vi "Main.vi"() -> ()   [LabVIEW 2021] (continued)
                    n838 = invoke on="控件配置文件" class="Tbl (严格)" method="Set Cell Value"("X Index"=0 ("X索引"), "Y Index"=w1041, "Value"=w1046) -> ()  [unwired: 3 in, 6 out]
                  }
                  frame "关联到曲线29" {
                    w1052 = T9 58 items=["刷新间隔", "波特率", "布尔1设置项", "布尔2设置项", "布尔3设置项", "布尔4设置项", "布尔5设置项", "布尔6设置项", "布尔7设置项", "布尔8设置项", "显控1设置", "显控2设置", "显控3设置", "显控4设置", "显控5设置", "显控6设置", "显控7设置", "显控8设置", "显控9设置", "显控10设置", "显控11设置", "显控12设置", "设控1设置", "设控2设置", "设控3设置", "设控4设置", "设控5设置", "设控6设置", "设控7设置", "设控8设置", "曲线1设置", "曲线2设置", "曲线3设置", "曲线4设置", "曲线5设置", "曲线6设置", "曲线7设置", "曲线8设置", "曲线9设置", "曲线10设置", "曲线11设置", "曲线12设置", "曲线13设置", "曲线14设置", "曲线15设置", "曲线16设置", "曲线17设置", "曲线18设置", "曲线19设置", "曲线20设置", "曲线21设置", "曲线22设置", "曲线23设置", "曲线24设置", "曲线25设置", "曲线26设置", "曲线27设置", "曲线28设置", "曲线29设置", "曲线30设置", "曲线31设置", "曲线32设置", "曲线33设置", "曲线34设置", "曲线35设置", "曲线36设置", "曲线37设置", "曲线38设置", "曲线39设置", "曲线40设置", "曲线41设置", "曲线42设置", "曲线43设置", "曲线44设置", "曲线45设置", "曲线46设置", "曲线47设置", "曲线48设置", "曲线49设置", "曲线50设置", "曲线51设置", "曲线52设置", "曲线53设置", "曲线54设置", "曲线55设置", "曲线56设置", "曲线57设置", "曲线58设置", "曲线59设置", "曲线60设置", "曲线61设置", "曲线62设置", "曲线63设置", "曲线64设置", "ID值", "数据模式"] ("DataInitDef")
                    n839 = property on="表格" class="Tbl (严格)"() -> ("Selection Start"=w1062:T1)  [unwired: 2 in, 2 out]
                    n840 = Unbundle By Name(w1062) -> ("Row"=w1060:i32)
                    n841 = property on="表格" class="Tbl (严格)"() -> ("Value"=w1061:string[][])  [unwired: 2 in, 2 out]
                    n842 = Number To Decimal String(number=w1060) -> (decimal integer string=w1059:string)  [unwired: 1 in]
                    n843 = Index Array(array=w1061, index (row)=w1060, index (col)=0 ("禁用的索引 (列)")) -> (element=w1058:string)
                    n844 = String Subset(string=w1058, length (rest)=16 ("长度（剩余）")) -> (substring=w1057:string)  [unwired: 1 in]
                    n845 = property on="曲线29设置" class="Str"("Val(Sgnl)"=w1057) -> ()  [unwired: 2 in, 2 out]
                    n846 = invoke on="控件配置文件" class="Tbl (严格)" method="Set Cell Value"("X Index"=1 ("X索引"), "Y Index"=w1052, "Value"=w1059) -> ()  [unwired: 3 in, 6 out]
                    n847 = invoke on="控件配置文件" class="Tbl (严格)" method="Set Cell Value"("X Index"=0 ("X索引"), "Y Index"=w1052, "Value"=w1057) -> ()  [unwired: 3 in, 6 out]
                  }
                  frame "关联到曲线30" {
                    w1063 = T9 59 items=["刷新间隔", "波特率", "布尔1设置项", "布尔2设置项", "布尔3设置项", "布尔4设置项", "布尔5设置项", "布尔6设置项", "布尔7设置项", "布尔8设置项", "显控1设置", "显控2设置", "显控3设置", "显控4设置", "显控5设置", "显控6设置", "显控7设置", "显控8设置", "显控9设置", "显控10设置", "显控11设置", "显控12设置", "设控1设置", "设控2设置", "设控3设置", "设控4设置", "设控5设置", "设控6设置", "设控7设置", "设控8设置", "曲线1设置", "曲线2设置", "曲线3设置", "曲线4设置", "曲线5设置", "曲线6设置", "曲线7设置", "曲线8设置", "曲线9设置", "曲线10设置", "曲线11设置", "曲线12设置", "曲线13设置", "曲线14设置", "曲线15设置", "曲线16设置", "曲线17设置", "曲线18设置", "曲线19设置", "曲线20设置", "曲线21设置", "曲线22设置", "曲线23设置", "曲线24设置", "曲线25设置", "曲线26设置", "曲线27设置", "曲线28设置", "曲线29设置", "曲线30设置", "曲线31设置", "曲线32设置", "曲线33设置", "曲线34设置", "曲线35设置", "曲线36设置", "曲线37设置", "曲线38设置", "曲线39设置", "曲线40设置", "曲线41设置", "曲线42设置", "曲线43设置", "曲线44设置", "曲线45设置", "曲线46设置", "曲线47设置", "曲线48设置", "曲线49设置", "曲线50设置", "曲线51设置", "曲线52设置", "曲线53设置", "曲线54设置", "曲线55设置", "曲线56设置", "曲线57设置", "曲线58设置", "曲线59设置", "曲线60设置", "曲线61设置", "曲线62设置", "曲线63设置", "曲线64设置", "ID值", "数据模式"] ("DataInitDef")
                    n848 = property on="表格" class="Tbl (严格)"() -> ("Selection Start"=w1073:T1)  [unwired: 2 in, 2 out]
                    n849 = Unbundle By Name(w1073) -> ("Row"=w1071:i32)
                    n850 = property on="表格" class="Tbl (严格)"() -> ("Value"=w1072:string[][])  [unwired: 2 in, 2 out]
                    n851 = Number To Decimal String(number=w1071) -> (decimal integer string=w1070:string)  [unwired: 1 in]
                    n852 = Index Array(array=w1072, index (row)=w1071, index (col)=0 ("禁用的索引 (列)")) -> (element=w1069:string)
                    n853 = String Subset(string=w1069, length (rest)=16 ("长度（剩余）")) -> (substring=w1068:string)  [unwired: 1 in]
                    n854 = property on="曲线30设置" class="Str"("Val(Sgnl)"=w1068) -> ()  [unwired: 2 in, 2 out]
                    n855 = invoke on="控件配置文件" class="Tbl (严格)" method="Set Cell Value"("X Index"=1 ("X索引"), "Y Index"=w1063, "Value"=w1070) -> ()  [unwired: 3 in, 6 out]
                    n856 = invoke on="控件配置文件" class="Tbl (严格)" method="Set Cell Value"("X Index"=0 ("X索引"), "Y Index"=w1063, "Value"=w1068) -> ()  [unwired: 3 in, 6 out]
                  }
                  frame "关联到曲线31" {
                    w1074 = T9 60 items=["刷新间隔", "波特率", "布尔1设置项", "布尔2设置项", "布尔3设置项", "布尔4设置项", "布尔5设置项", "布尔6设置项", "布尔7设置项", "布尔8设置项", "显控1设置", "显控2设置", "显控3设置", "显控4设置", "显控5设置", "显控6设置", "显控7设置", "显控8设置", "显控9设置", "显控10设置", "显控11设置", "显控12设置", "设控1设置", "设控2设置", "设控3设置", "设控4设置", "设控5设置", "设控6设置", "设控7设置", "设控8设置", "曲线1设置", "曲线2设置", "曲线3设置", "曲线4设置", "曲线5设置", "曲线6设置", "曲线7设置", "曲线8设置", "曲线9设置", "曲线10设置", "曲线11设置", "曲线12设置", "曲线13设置", "曲线14设置", "曲线15设置", "曲线16设置", "曲线17设置", "曲线18设置", "曲线19设置", "曲线20设置", "曲线21设置", "曲线22设置", "曲线23设置", "曲线24设置", "曲线25设置", "曲线26设置", "曲线27设置", "曲线28设置", "曲线29设置", "曲线30设置", "曲线31设置", "曲线32设置", "曲线33设置", "曲线34设置", "曲线35设置", "曲线36设置", "曲线37设置", "曲线38设置", "曲线39设置", "曲线40设置", "曲线41设置", "曲线42设置", "曲线43设置", "曲线44设置", "曲线45设置", "曲线46设置", "曲线47设置", "曲线48设置", "曲线49设置", "曲线50设置", "曲线51设置", "曲线52设置", "曲线53设置", "曲线54设置", "曲线55设置", "曲线56设置", "曲线57设置", "曲线58设置", "曲线59设置", "曲线60设置", "曲线61设置", "曲线62设置", "曲线63设置", "曲线64设置", "ID值", "数据模式"] ("DataInitDef")
                    n857 = property on="表格" class="Tbl (严格)"() -> ("Selection Start"=w1084:T1)  [unwired: 2 in, 2 out]
                    n858 = Unbundle By Name(w1084) -> ("Row"=w1082:i32)
                    n859 = property on="表格" class="Tbl (严格)"() -> ("Value"=w1083:string[][])  [unwired: 2 in, 2 out]
                    n860 = Number To Decimal String(number=w1082) -> (decimal integer string=w1081:string)  [unwired: 1 in]
                    n861 = Index Array(array=w1083, index (row)=w1082, index (col)=0 ("禁用的索引 (列)")) -> (element=w1080:string)
                    n862 = String Subset(string=w1080, length (rest)=16 ("长度（剩余）")) -> (substring=w1079:string)  [unwired: 1 in]
                    n863 = property on="曲线31设置" class="Str"("Val(Sgnl)"=w1079) -> ()  [unwired: 2 in, 2 out]
                    n864 = invoke on="控件配置文件" class="Tbl (严格)" method="Set Cell Value"("X Index"=1 ("X索引"), "Y Index"=w1074, "Value"=w1081) -> ()  [unwired: 3 in, 6 out]
                    n865 = invoke on="控件配置文件" class="Tbl (严格)" method="Set Cell Value"("X Index"=0 ("X索引"), "Y Index"=w1074, "Value"=w1079) -> ()  [unwired: 3 in, 6 out]
                  }
                  frame "关联到曲线32" {
                    w1085 = T9 61 items=["刷新间隔", "波特率", "布尔1设置项", "布尔2设置项", "布尔3设置项", "布尔4设置项", "布尔5设置项", "布尔6设置项", "布尔7设置项", "布尔8设置项", "显控1设置", "显控2设置", "显控3设置", "显控4设置", "显控5设置", "显控6设置", "显控7设置", "显控8设置", "显控9设置", "显控10设置", "显控11设置", "显控12设置", "设控1设置", "设控2设置", "设控3设置", "设控4设置", "设控5设置", "设控6设置", "设控7设置", "设控8设置", "曲线1设置", "曲线2设置", "曲线3设置", "曲线4设置", "曲线5设置", "曲线6设置", "曲线7设置", "曲线8设置", "曲线9设置", "曲线10设置", "曲线11设置", "曲线12设置", "曲线13设置", "曲线14设置", "曲线15设置", "曲线16设置", "曲线17设置", "曲线18设置", "曲线19设置", "曲线20设置", "曲线21设置", "曲线22设置", "曲线23设置", "曲线24设置", "曲线25设置", "曲线26设置", "曲线27设置", "曲线28设置", "曲线29设置", "曲线30设置", "曲线31设置", "曲线32设置", "曲线33设置", "曲线34设置", "曲线35设置", "曲线36设置", "曲线37设置", "曲线38设置", "曲线39设置", "曲线40设置", "曲线41设置", "曲线42设置", "曲线43设置", "曲线44设置", "曲线45设置", "曲线46设置", "曲线47设置", "曲线48设置", "曲线49设置", "曲线50设置", "曲线51设置", "曲线52设置", "曲线53设置", "曲线54设置", "曲线55设置", "曲线56设置", "曲线57设置", "曲线58设置", "曲线59设置", "曲线60设置", "曲线61设置", "曲线62设置", "曲线63设置", "曲线64设置", "ID值", "数据模式"] ("DataInitDef")
                    n866 = property on="表格" class="Tbl (严格)"() -> ("Selection Start"=w1095:T1)  [unwired: 2 in, 2 out]
                    n867 = Unbundle By Name(w1095) -> ("Row"=w1093:i32)
                    n868 = property on="表格" class="Tbl (严格)"() -> ("Value"=w1094:string[][])  [unwired: 2 in, 2 out]
                    n869 = Number To Decimal String(number=w1093) -> (decimal integer string=w1092:string)  [unwired: 1 in]
                    n870 = Index Array(array=w1094, index (row)=w1093, index (col)=0 ("禁用的索引 (列)")) -> (element=w1091:string)
                    n871 = String Subset(string=w1091, length (rest)=16 ("长度（剩余）")) -> (substring=w1090:string)  [unwired: 1 in]
                    n872 = property on="曲线32设置" class="Str"("Val(Sgnl)"=w1090) -> ()  [unwired: 2 in, 2 out]
                    n873 = invoke on="控件配置文件" class="Tbl (严格)" method="Set Cell Value"("X Index"=1 ("X索引"), "Y Index"=w1085, "Value"=w1092) -> ()  [unwired: 3 in, 6 out]
                    n874 = invoke on="控件配置文件" class="Tbl (严格)" method="Set Cell Value"("X Index"=0 ("X索引"), "Y Index"=w1085, "Value"=w1090) -> ()  [unwired: 3 in, 6 out]
                  }
                  frame "关联到曲线33" {
                    w1096 = T9 62 items=["刷新间隔", "波特率", "布尔1设置项", "布尔2设置项", "布尔3设置项", "布尔4设置项", "布尔5设置项", "布尔6设置项", "布尔7设置项", "布尔8设置项", "显控1设置", "显控2设置", "显控3设置", "显控4设置", "显控5设置", "显控6设置", "显控7设置", "显控8设置", "显控9设置", "显控10设置", "显控11设置", "显控12设置", "设控1设置", "设控2设置", "设控3设置", "设控4设置", "设控5设置", "设控6设置", "设控7设置", "设控8设置", "曲线1设置", "曲线2设置", "曲线3设置", "曲线4设置", "曲线5设置", "曲线6设置", "曲线7设置", "曲线8设置", "曲线9设置", "曲线10设置", "曲线11设置", "曲线12设置", "曲线13设置", "曲线14设置", "曲线15设置", "曲线16设置", "曲线17设置", "曲线18设置", "曲线19设置", "曲线20设置", "曲线21设置", "曲线22设置", "曲线23设置", "曲线24设置", "曲线25设置", "曲线26设置", "曲线27设置", "曲线28设置", "曲线29设置", "曲线30设置", "曲线31设置", "曲线32设置", "曲线33设置", "曲线34设置", "曲线35设置", "曲线36设置", "曲线37设置", "曲线38设置", "曲线39设置", "曲线40设置", "曲线41设置", "曲线42设置", "曲线43设置", "曲线44设置", "曲线45设置", "曲线46设置", "曲线47设置", "曲线48设置", "曲线49设置", "曲线50设置", "曲线51设置", "曲线52设置", "曲线53设置", "曲线54设置", "曲线55设置", "曲线56设置", "曲线57设置", "曲线58设置", "曲线59设置", "曲线60设置", "曲线61设置", "曲线62设置", "曲线63设置", "曲线64设置", "ID值", "数据模式"] ("DataInitDef")
                    n875 = property on="表格" class="Tbl (严格)"() -> ("Selection Start"=w1106:T1)  [unwired: 2 in, 2 out]
                    n876 = Unbundle By Name(w1106) -> ("Row"=w1104:i32)
                    n877 = property on="表格" class="Tbl (严格)"() -> ("Value"=w1105:string[][])  [unwired: 2 in, 2 out]
                    n878 = Number To Decimal String(number=w1104) -> (decimal integer string=w1103:string)  [unwired: 1 in]
                    n879 = Index Array(array=w1105, index (row)=w1104, index (col)=0 ("禁用的索引 (列)")) -> (element=w1102:string)
                    n880 = String Subset(string=w1102, length (rest)=16 ("长度（剩余）")) -> (substring=w1101:string)  [unwired: 1 in]
                    n881 = property on="曲线33设置" class="Str"("Val(Sgnl)"=w1101) -> ()  [unwired: 2 in, 2 out]
                    n882 = invoke on="控件配置文件" class="Tbl (严格)" method="Set Cell Value"("X Index"=1 ("X索引"), "Y Index"=w1096, "Value"=w1103) -> ()  [unwired: 3 in, 6 out]
                    n883 = invoke on="控件配置文件" class="Tbl (严格)" method="Set Cell Value"("X Index"=0 ("X索引"), "Y Index"=w1096, "Value"=w1101) -> ()  [unwired: 3 in, 6 out]
                  }
                  frame "关联到曲线34" {
                    w1107 = T9 63 items=["刷新间隔", "波特率", "布尔1设置项", "布尔2设置项", "布尔3设置项", "布尔4设置项", "布尔5设置项", "布尔6设置项", "布尔7设置项", "布尔8设置项", "显控1设置", "显控2设置", "显控3设置", "显控4设置", "显控5设置", "显控6设置", "显控7设置", "显控8设置", "显控9设置", "显控10设置", "显控11设置", "显控12设置", "设控1设置", "设控2设置", "设控3设置", "设控4设置", "设控5设置", "设控6设置", "设控7设置", "设控8设置", "曲线1设置", "曲线2设置", "曲线3设置", "曲线4设置", "曲线5设置", "曲线6设置", "曲线7设置", "曲线8设置", "曲线9设置", "曲线10设置", "曲线11设置", "曲线12设置", "曲线13设置", "曲线14设置", "曲线15设置", "曲线16设置", "曲线17设置", "曲线18设置", "曲线19设置", "曲线20设置", "曲线21设置", "曲线22设置", "曲线23设置", "曲线24设置", "曲线25设置", "曲线26设置", "曲线27设置", "曲线28设置", "曲线29设置", "曲线30设置", "曲线31设置", "曲线32设置", "曲线33设置", "曲线34设置", "曲线35设置", "曲线36设置", "曲线37设置", "曲线38设置", "曲线39设置", "曲线40设置", "曲线41设置", "曲线42设置", "曲线43设置", "曲线44设置", "曲线45设置", "曲线46设置", "曲线47设置", "曲线48设置", "曲线49设置", "曲线50设置", "曲线51设置", "曲线52设置", "曲线53设置", "曲线54设置", "曲线55设置", "曲线56设置", "曲线57设置", "曲线58设置", "曲线59设置", "曲线60设置", "曲线61设置", "曲线62设置", "曲线63设置", "曲线64设置", "ID值", "数据模式"] ("DataInitDef")
                    n884 = property on="表格" class="Tbl (严格)"() -> ("Selection Start"=w1117:T1)  [unwired: 2 in, 2 out]
                    n885 = Unbundle By Name(w1117) -> ("Row"=w1115:i32)
                    n886 = property on="表格" class="Tbl (严格)"() -> ("Value"=w1116:string[][])  [unwired: 2 in, 2 out]
                    n887 = Number To Decimal String(number=w1115) -> (decimal integer string=w1114:string)  [unwired: 1 in]
                    n888 = Index Array(array=w1116, index (row)=w1115, index (col)=0 ("禁用的索引 (列)")) -> (element=w1113:string)
                    n889 = String Subset(string=w1113, length (rest)=16 ("长度（剩余）")) -> (substring=w1112:string)  [unwired: 1 in]
                    n890 = property on="曲线34设置" class="Str"("Val(Sgnl)"=w1112) -> ()  [unwired: 2 in, 2 out]
                    n891 = invoke on="控件配置文件" class="Tbl (严格)" method="Set Cell Value"("X Index"=1 ("X索引"), "Y Index"=w1107, "Value"=w1114) -> ()  [unwired: 3 in, 6 out]
                    n892 = invoke on="控件配置文件" class="Tbl (严格)" method="Set Cell Value"("X Index"=0 ("X索引"), "Y Index"=w1107, "Value"=w1112) -> ()  [unwired: 3 in, 6 out]
                  }
                  frame "关联到曲线35" {
                    w1118 = T9 64 items=["刷新间隔", "波特率", "布尔1设置项", "布尔2设置项", "布尔3设置项", "布尔4设置项", "布尔5设置项", "布尔6设置项", "布尔7设置项", "布尔8设置项", "显控1设置", "显控2设置", "显控3设置", "显控4设置", "显控5设置", "显控6设置", "显控7设置", "显控8设置", "显控9设置", "显控10设置", "显控11设置", "显控12设置", "设控1设置", "设控2设置", "设控3设置", "设控4设置", "设控5设置", "设控6设置", "设控7设置", "设控8设置", "曲线1设置", "曲线2设置", "曲线3设置", "曲线4设置", "曲线5设置", "曲线6设置", "曲线7设置", "曲线8设置", "曲线9设置", "曲线10设置", "曲线11设置", "曲线12设置", "曲线13设置", "曲线14设置", "曲线15设置", "曲线16设置", "曲线17设置", "曲线18设置", "曲线19设置", "曲线20设置", "曲线21设置", "曲线22设置", "曲线23设置", "曲线24设置", "曲线25设置", "曲线26设置", "曲线27设置", "曲线28设置", "曲线29设置", "曲线30设置", "曲线31设置", "曲线32设置", "曲线33设置", "曲线34设置", "曲线35设置", "曲线36设置", "曲线37设置", "曲线38设置", "曲线39设置", "曲线40设置", "曲线41设置", "曲线42设置", "曲线43设置", "曲线44设置", "曲线45设置", "曲线46设置", "曲线47设置", "曲线48设置", "曲线49设置", "曲线50设置", "曲线51设置", "曲线52设置", "曲线53设置", "曲线54设置", "曲线55设置", "曲线56设置", "曲线57设置", "曲线58设置", "曲线59设置", "曲线60设置", "曲线61设置", "曲线62设置", "曲线63设置", "曲线64设置", "ID值", "数据模式"] ("DataInitDef")
                    n893 = property on="表格" class="Tbl (严格)"() -> ("Selection Start"=w1128:T1)  [unwired: 2 in, 2 out]
                    n894 = Unbundle By Name(w1128) -> ("Row"=w1126:i32)
                    n895 = property on="表格" class="Tbl (严格)"() -> ("Value"=w1127:string[][])  [unwired: 2 in, 2 out]
                    n896 = Number To Decimal String(number=w1126) -> (decimal integer string=w1125:string)  [unwired: 1 in]
                    n897 = Index Array(array=w1127, index (row)=w1126, index (col)=0 ("禁用的索引 (列)")) -> (element=w1124:string)
                    n898 = String Subset(string=w1124, length (rest)=16 ("长度（剩余）")) -> (substring=w1123:string)  [unwired: 1 in]
                    n899 = property on="曲线35设置" class="Str"("Val(Sgnl)"=w1123) -> ()  [unwired: 2 in, 2 out]
                    n900 = invoke on="控件配置文件" class="Tbl (严格)" method="Set Cell Value"("X Index"=1 ("X索引"), "Y Index"=w1118, "Value"=w1125) -> ()  [unwired: 3 in, 6 out]
                    n901 = invoke on="控件配置文件" class="Tbl (严格)" method="Set Cell Value"("X Index"=0 ("X索引"), "Y Index"=w1118, "Value"=w1123) -> ()  [unwired: 3 in, 6 out]
                  }
                  frame "关联到曲线36" {
                    w1129 = T9 65 items=["刷新间隔", "波特率", "布尔1设置项", "布尔2设置项", "布尔3设置项", "布尔4设置项", "布尔5设置项", "布尔6设置项", "布尔7设置项", "布尔8设置项", "显控1设置", "显控2设置", "显控3设置", "显控4设置", "显控5设置", "显控6设置", "显控7设置", "显控8设置", "显控9设置", "显控10设置", "显控11设置", "显控12设置", "设控1设置", "设控2设置", "设控3设置", "设控4设置", "设控5设置", "设控6设置", "设控7设置", "设控8设置", "曲线1设置", "曲线2设置", "曲线3设置", "曲线4设置", "曲线5设置", "曲线6设置", "曲线7设置", "曲线8设置", "曲线9设置", "曲线10设置", "曲线11设置", "曲线12设置", "曲线13设置", "曲线14设置", "曲线15设置", "曲线16设置", "曲线17设置", "曲线18设置", "曲线19设置", "曲线20设置", "曲线21设置", "曲线22设置", "曲线23设置", "曲线24设置", "曲线25设置", "曲线26设置", "曲线27设置", "曲线28设置", "曲线29设置", "曲线30设置", "曲线31设置", "曲线32设置", "曲线33设置", "曲线34设置", "曲线35设置", "曲线36设置", "曲线37设置", "曲线38设置", "曲线39设置", "曲线40设置", "曲线41设置", "曲线42设置", "曲线43设置", "曲线44设置", "曲线45设置", "曲线46设置", "曲线47设置", "曲线48设置", "曲线49设置", "曲线50设置", "曲线51设置", "曲线52设置", "曲线53设置", "曲线54设置", "曲线55设置", "曲线56设置", "曲线57设置", "曲线58设置", "曲线59设置", "曲线60设置", "曲线61设置", "曲线62设置", "曲线63设置", "曲线64设置", "ID值", "数据模式"] ("DataInitDef")
                    n902 = property on="表格" class="Tbl (严格)"() -> ("Selection Start"=w1139:T1)  [unwired: 2 in, 2 out]
                    n903 = Unbundle By Name(w1139) -> ("Row"=w1137:i32)
                    n904 = property on="表格" class="Tbl (严格)"() -> ("Value"=w1138:string[][])  [unwired: 2 in, 2 out]
                    n905 = Number To Decimal String(number=w1137) -> (decimal integer string=w1136:string)  [unwired: 1 in]
                    n906 = Index Array(array=w1138, index (row)=w1137, index (col)=0 ("禁用的索引 (列)")) -> (element=w1135:string)
                    n907 = String Subset(string=w1135, length (rest)=16 ("长度（剩余）")) -> (substring=w1134:string)  [unwired: 1 in]
                    n908 = property on="曲线36设置" class="Str"("Val(Sgnl)"=w1134) -> ()  [unwired: 2 in, 2 out]
                    n909 = invoke on="控件配置文件" class="Tbl (严格)" method="Set Cell Value"("X Index"=1 ("X索引"), "Y Index"=w1129, "Value"=w1136) -> ()  [unwired: 3 in, 6 out]
                    n910 = invoke on="控件配置文件" class="Tbl (严格)" method="Set Cell Value"("X Index"=0 ("X索引"), "Y Index"=w1129, "Value"=w1134) -> ()  [unwired: 3 in, 6 out]
                  }
                  frame "关联到曲线37" {
                    w1140 = T9 66 items=["刷新间隔", "波特率", "布尔1设置项", "布尔2设置项", "布尔3设置项", "布尔4设置项", "布尔5设置项", "布尔6设置项", "布尔7设置项", "布尔8设置项", "显控1设置", "显控2设置", "显控3设置", "显控4设置", "显控5设置", "显控6设置", "显控7设置", "显控8设置", "显控9设置", "显控10设置", "显控11设置", "显控12设置", "设控1设置", "设控2设置", "设控3设置", "设控4设置", "设控5设置", "设控6设置", "设控7设置", "设控8设置", "曲线1设置", "曲线2设置", "曲线3设置", "曲线4设置", "曲线5设置", "曲线6设置", "曲线7设置", "曲线8设置", "曲线9设置", "曲线10设置", "曲线11设置", "曲线12设置", "曲线13设置", "曲线14设置", "曲线15设置", "曲线16设置", "曲线17设置", "曲线18设置", "曲线19设置", "曲线20设置", "曲线21设置", "曲线22设置", "曲线23设置", "曲线24设置", "曲线25设置", "曲线26设置", "曲线27设置", "曲线28设置", "曲线29设置", "曲线30设置", "曲线31设置", "曲线32设置", "曲线33设置", "曲线34设置", "曲线35设置", "曲线36设置", "曲线37设置", "曲线38设置", "曲线39设置", "曲线40设置", "曲线41设置", "曲线42设置", "曲线43设置", "曲线44设置", "曲线45设置", "曲线46设置", "曲线47设置", "曲线48设置", "曲线49设置", "曲线50设置", "曲线51设置", "曲线52设置", "曲线53设置", "曲线54设置", "曲线55设置", "曲线56设置", "曲线57设置", "曲线58设置", "曲线59设置", "曲线60设置", "曲线61设置", "曲线62设置", "曲线63设置", "曲线64设置", "ID值", "数据模式"] ("DataInitDef")
                    n911 = property on="表格" class="Tbl (严格)"() -> ("Selection Start"=w1150:T1)  [unwired: 2 in, 2 out]
                    n912 = Unbundle By Name(w1150) -> ("Row"=w1148:i32)
                    n913 = property on="表格" class="Tbl (严格)"() -> ("Value"=w1149:string[][])  [unwired: 2 in, 2 out]
                    n914 = Number To Decimal String(number=w1148) -> (decimal integer string=w1147:string)  [unwired: 1 in]
                    n915 = Index Array(array=w1149, index (row)=w1148, index (col)=0 ("禁用的索引 (列)")) -> (element=w1146:string)
                    n916 = String Subset(string=w1146, length (rest)=16 ("长度（剩余）")) -> (substring=w1145:string)  [unwired: 1 in]
                    n917 = property on="曲线37设置" class="Str"("Val(Sgnl)"=w1145) -> ()  [unwired: 2 in, 2 out]
                    n918 = invoke on="控件配置文件" class="Tbl (严格)" method="Set Cell Value"("X Index"=1 ("X索引"), "Y Index"=w1140, "Value"=w1147) -> ()  [unwired: 3 in, 6 out]
                    n919 = invoke on="控件配置文件" class="Tbl (严格)" method="Set Cell Value"("X Index"=0 ("X索引"), "Y Index"=w1140, "Value"=w1145) -> ()  [unwired: 3 in, 6 out]
                  }
                  frame "关联到曲线38" {
                    w1151 = T9 67 items=["刷新间隔", "波特率", "布尔1设置项", "布尔2设置项", "布尔3设置项", "布尔4设置项", "布尔5设置项", "布尔6设置项", "布尔7设置项", "布尔8设置项", "显控1设置", "显控2设置", "显控3设置", "显控4设置", "显控5设置", "显控6设置", "显控7设置", "显控8设置", "显控9设置", "显控10设置", "显控11设置", "显控12设置", "设控1设置", "设控2设置", "设控3设置", "设控4设置", "设控5设置", "设控6设置", "设控7设置", "设控8设置", "曲线1设置", "曲线2设置", "曲线3设置", "曲线4设置", "曲线5设置", "曲线6设置", "曲线7设置", "曲线8设置", "曲线9设置", "曲线10设置", "曲线11设置", "曲线12设置", "曲线13设置", "曲线14设置", "曲线15设置", "曲线16设置", "曲线17设置", "曲线18设置", "曲线19设置", "曲线20设置", "曲线21设置", "曲线22设置", "曲线23设置", "曲线24设置", "曲线25设置", "曲线26设置", "曲线27设置", "曲线28设置", "曲线29设置", "曲线30设置", "曲线31设置", "曲线32设置", "曲线33设置", "曲线34设置", "曲线35设置", "曲线36设置", "曲线37设置", "曲线38设置", "曲线39设置", "曲线40设置", "曲线41设置", "曲线42设置", "曲线43设置", "曲线44设置", "曲线45设置", "曲线46设置", "曲线47设置", "曲线48设置", "曲线49设置", "曲线50设置", "曲线51设置", "曲线52设置", "曲线53设置", "曲线54设置", "曲线55设置", "曲线56设置", "曲线57设置", "曲线58设置", "曲线59设置", "曲线60设置", "曲线61设置", "曲线62设置", "曲线63设置", "曲线64设置", "ID值", "数据模式"] ("DataInitDef")
                    n920 = property on="表格" class="Tbl (严格)"() -> ("Selection Start"=w1161:T1)  [unwired: 2 in, 2 out]
                    n921 = Unbundle By Name(w1161) -> ("Row"=w1159:i32)
                    n922 = property on="表格" class="Tbl (严格)"() -> ("Value"=w1160:string[][])  [unwired: 2 in, 2 out]
                    n923 = Number To Decimal String(number=w1159) -> (decimal integer string=w1158:string)  [unwired: 1 in]
                    n924 = Index Array(array=w1160, index (row)=w1159, index (col)=0 ("禁用的索引 (列)")) -> (element=w1157:string)
                    n925 = String Subset(string=w1157, length (rest)=16 ("长度（剩余）")) -> (substring=w1156:string)  [unwired: 1 in]
                    n926 = property on="曲线38设置" class="Str"("Val(Sgnl)"=w1156) -> ()  [unwired: 2 in, 2 out]
                    n927 = invoke on="控件配置文件" class="Tbl (严格)" method="Set Cell Value"("X Index"=1 ("X索引"), "Y Index"=w1151, "Value"=w1158) -> ()  [unwired: 3 in, 6 out]
                    n928 = invoke on="控件配置文件" class="Tbl (严格)" method="Set Cell Value"("X Index"=0 ("X索引"), "Y Index"=w1151, "Value"=w1156) -> ()  [unwired: 3 in, 6 out]
                  }
                  frame "关联到曲线39" {
                    w1162 = T9 68 items=["刷新间隔", "波特率", "布尔1设置项", "布尔2设置项", "布尔3设置项", "布尔4设置项", "布尔5设置项", "布尔6设置项", "布尔7设置项", "布尔8设置项", "显控1设置", "显控2设置", "显控3设置", "显控4设置", "显控5设置", "显控6设置", "显控7设置", "显控8设置", "显控9设置", "显控10设置", "显控11设置", "显控12设置", "设控1设置", "设控2设置", "设控3设置", "设控4设置", "设控5设置", "设控6设置", "设控7设置", "设控8设置", "曲线1设置", "曲线2设置", "曲线3设置", "曲线4设置", "曲线5设置", "曲线6设置", "曲线7设置", "曲线8设置", "曲线9设置", "曲线10设置", "曲线11设置", "曲线12设置", "曲线13设置", "曲线14设置", "曲线15设置", "曲线16设置", "曲线17设置", "曲线18设置", "曲线19设置", "曲线20设置", "曲线21设置", "曲线22设置", "曲线23设置", "曲线24设置", "曲线25设置", "曲线26设置", "曲线27设置", "曲线28设置", "曲线29设置", "曲线30设置", "曲线31设置", "曲线32设置", "曲线33设置", "曲线34设置", "曲线35设置", "曲线36设置", "曲线37设置", "曲线38设置", "曲线39设置", "曲线40设置", "曲线41设置", "曲线42设置", "曲线43设置", "曲线44设置", "曲线45设置", "曲线46设置", "曲线47设置", "曲线48设置", "曲线49设置", "曲线50设置", "曲线51设置", "曲线52设置", "曲线53设置", "曲线54设置", "曲线55设置", "曲线56设置", "曲线57设置", "曲线58设置", "曲线59设置", "曲线60设置", "曲线61设置", "曲线62设置", "曲线63设置", "曲线64设置", "ID值", "数据模式"] ("DataInitDef")
                    n929 = property on="表格" class="Tbl (严格)"() -> ("Selection Start"=w1172:T1)  [unwired: 2 in, 2 out]
                    n930 = Unbundle By Name(w1172) -> ("Row"=w1170:i32)
                    n931 = property on="表格" class="Tbl (严格)"() -> ("Value"=w1171:string[][])  [unwired: 2 in, 2 out]
                    n932 = Number To Decimal String(number=w1170) -> (decimal integer string=w1169:string)  [unwired: 1 in]
                    n933 = Index Array(array=w1171, index (row)=w1170, index (col)=0 ("禁用的索引 (列)")) -> (element=w1168:string)
                    n934 = String Subset(string=w1168, length (rest)=16 ("长度（剩余）")) -> (substring=w1167:string)  [unwired: 1 in]
                    n935 = property on="曲线39设置" class="Str"("Val(Sgnl)"=w1167) -> ()  [unwired: 2 in, 2 out]
                    n936 = invoke on="控件配置文件" class="Tbl (严格)" method="Set Cell Value"("X Index"=1 ("X索引"), "Y Index"=w1162, "Value"=w1169) -> ()  [unwired: 3 in, 6 out]
                    n937 = invoke on="控件配置文件" class="Tbl (严格)" method="Set Cell Value"("X Index"=0 ("X索引"), "Y Index"=w1162, "Value"=w1167) -> ()  [unwired: 3 in, 6 out]
                  }
                  frame "关联到曲线40" {
                    w1173 = T9 69 items=["刷新间隔", "波特率", "布尔1设置项", "布尔2设置项", "布尔3设置项", "布尔4设置项", "布尔5设置项", "布尔6设置项", "布尔7设置项", "布尔8设置项", "显控1设置", "显控2设置", "显控3设置", "显控4设置", "显控5设置", "显控6设置", "显控7设置", "显控8设置", "显控9设置", "显控10设置", "显控11设置", "显控12设置", "设控1设置", "设控2设置", "设控3设置", "设控4设置", "设控5设置", "设控6设置", "设控7设置", "设控8设置", "曲线1设置", "曲线2设置", "曲线3设置", "曲线4设置", "曲线5设置", "曲线6设置", "曲线7设置", "曲线8设置", "曲线9设置", "曲线10设置", "曲线11设置", "曲线12设置", "曲线13设置", "曲线14设置", "曲线15设置", "曲线16设置", "曲线17设置", "曲线18设置", "曲线19设置", "曲线20设置", "曲线21设置", "曲线22设置", "曲线23设置", "曲线24设置", "曲线25设置", "曲线26设置", "曲线27设置", "曲线28设置", "曲线29设置", "曲线30设置", "曲线31设置", "曲线32设置", "曲线33设置", "曲线34设置", "曲线35设置", "曲线36设置", "曲线37设置", "曲线38设置", "曲线39设置", "曲线40设置", "曲线41设置", "曲线42设置", "曲线43设置", "曲线44设置", "曲线45设置", "曲线46设置", "曲线47设置", "曲线48设置", "曲线49设置", "曲线50设置", "曲线51设置", "曲线52设置", "曲线53设置", "曲线54设置", "曲线55设置", "曲线56设置", "曲线57设置", "曲线58设置", "曲线59设置", "曲线60设置", "曲线61设置", "曲线62设置", "曲线63设置", "曲线64设置", "ID值", "数据模式"] ("DataInitDef")
                    n938 = property on="表格" class="Tbl (严格)"() -> ("Selection Start"=w1183:T1)  [unwired: 2 in, 2 out]
                    n939 = Unbundle By Name(w1183) -> ("Row"=w1181:i32)
                    n940 = property on="表格" class="Tbl (严格)"() -> ("Value"=w1182:string[][])  [unwired: 2 in, 2 out]
                    n941 = Number To Decimal String(number=w1181) -> (decimal integer string=w1180:string)  [unwired: 1 in]
                    n942 = Index Array(array=w1182, index (row)=w1181, index (col)=0 ("禁用的索引 (列)")) -> (element=w1179:string)
                    n943 = String Subset(string=w1179, length (rest)=16 ("长度（剩余）")) -> (substring=w1178:string)  [unwired: 1 in]
                    n944 = property on="曲线40设置" class="Str"("Val(Sgnl)"=w1178) -> ()  [unwired: 2 in, 2 out]
                    n945 = invoke on="控件配置文件" class="Tbl (严格)" method="Set Cell Value"("X Index"=1 ("X索引"), "Y Index"=w1173, "Value"=w1180) -> ()  [unwired: 3 in, 6 out]
                    n946 = invoke on="控件配置文件" class="Tbl (严格)" method="Set Cell Value"("X Index"=0 ("X索引"), "Y Index"=w1173, "Value"=w1178) -> ()  [unwired: 3 in, 6 out]
                  }
                  frame "关联到曲线41" {
                    w1184 = T9 70 items=["刷新间隔", "波特率", "布尔1设置项", "布尔2设置项", "布尔3设置项", "布尔4设置项", "布尔5设置项", "布尔6设置项", "布尔7设置项", "布尔8设置项", "显控1设置", "显控2设置", "显控3设置", "显控4设置", "显控5设置", "显控6设置", "显控7设置", "显控8设置", "显控9设置", "显控10设置", "显控11设置", "显控12设置", "设控1设置", "设控2设置", "设控3设置", "设控4设置", "设控5设置", "设控6设置", "设控7设置", "设控8设置", "曲线1设置", "曲线2设置", "曲线3设置", "曲线4设置", "曲线5设置", "曲线6设置", "曲线7设置", "曲线8设置", "曲线9设置", "曲线10设置", "曲线11设置", "曲线12设置", "曲线13设置", "曲线14设置", "曲线15设置", "曲线16设置", "曲线17设置", "曲线18设置", "曲线19设置", "曲线20设置", "曲线21设置", "曲线22设置", "曲线23设置", "曲线24设置", "曲线25设置", "曲线26设置", "曲线27设置", "曲线28设置", "曲线29设置", "曲线30设置", "曲线31设置", "曲线32设置", "曲线33设置", "曲线34设置", "曲线35设置", "曲线36设置", "曲线37设置", "曲线38设置", "曲线39设置", "曲线40设置", "曲线41设置", "曲线42设置", "曲线43设置", "曲线44设置", "曲线45设置", "曲线46设置", "曲线47设置", "曲线48设置", "曲线49设置", "曲线50设置", "曲线51设置", "曲线52设置", "曲线53设置", "曲线54设置", "曲线55设置", "曲线56设置", "曲线57设置", "曲线58设置", "曲线59设置", "曲线60设置", "曲线61设置", "曲线62设置", "曲线63设置", "曲线64设置", "ID值", "数据模式"] ("DataInitDef")
                    n947 = property on="表格" class="Tbl (严格)"() -> ("Selection Start"=w1194:T1)  [unwired: 2 in, 2 out]
                    n948 = Unbundle By Name(w1194) -> ("Row"=w1192:i32)
                    n949 = property on="表格" class="Tbl (严格)"() -> ("Value"=w1193:string[][])  [unwired: 2 in, 2 out]
                    n950 = Number To Decimal String(number=w1192) -> (decimal integer string=w1191:string)  [unwired: 1 in]
                    n951 = Index Array(array=w1193, index (row)=w1192, index (col)=0 ("禁用的索引 (列)")) -> (element=w1190:string)
                    n952 = String Subset(string=w1190, length (rest)=16 ("长度（剩余）")) -> (substring=w1189:string)  [unwired: 1 in]
                    n953 = property on="曲线41设置" class="Str"("Val(Sgnl)"=w1189) -> ()  [unwired: 2 in, 2 out]
                    n954 = invoke on="控件配置文件" class="Tbl (严格)" method="Set Cell Value"("X Index"=1 ("X索引"), "Y Index"=w1184, "Value"=w1191) -> ()  [unwired: 3 in, 6 out]
                    n955 = invoke on="控件配置文件" class="Tbl (严格)" method="Set Cell Value"("X Index"=0 ("X索引"), "Y Index"=w1184, "Value"=w1189) -> ()  [unwired: 3 in, 6 out]
                  }
                  frame "关联到曲线42" {
                    w1195 = T9 71 items=["刷新间隔", "波特率", "布尔1设置项", "布尔2设置项", "布尔3设置项", "布尔4设置项", "布尔5设置项", "布尔6设置项", "布尔7设置项", "布尔8设置项", "显控1设置", "显控2设置", "显控3设置", "显控4设置", "显控5设置", "显控6设置", "显控7设置", "显控8设置", "显控9设置", "显控10设置", "显控11设置", "显控12设置", "设控1设置", "设控2设置", "设控3设置", "设控4设置", "设控5设置", "设控6设置", "设控7设置", "设控8设置", "曲线1设置", "曲线2设置", "曲线3设置", "曲线4设置", "曲线5设置", "曲线6设置", "曲线7设置", "曲线8设置", "曲线9设置", "曲线10设置", "曲线11设置", "曲线12设置", "曲线13设置", "曲线14设置", "曲线15设置", "曲线16设置", "曲线17设置", "曲线18设置", "曲线19设置", "曲线20设置", "曲线21设置", "曲线22设置", "曲线23设置", "曲线24设置", "曲线25设置", "曲线26设置", "曲线27设置", "曲线28设置", "曲线29设置", "曲线30设置", "曲线31设置", "曲线32设置", "曲线33设置", "曲线34设置", "曲线35设置", "曲线36设置", "曲线37设置", "曲线38设置", "曲线39设置", "曲线40设置", "曲线41设置", "曲线42设置", "曲线43设置", "曲线44设置", "曲线45设置", "曲线46设置", "曲线47设置", "曲线48设置", "曲线49设置", "曲线50设置", "曲线51设置", "曲线52设置", "曲线53设置", "曲线54设置", "曲线55设置", "曲线56设置", "曲线57设置", "曲线58设置", "曲线59设置", "曲线60设置", "曲线61设置", "曲线62设置", "曲线63设置", "曲线64设置", "ID值", "数据模式"] ("DataInitDef")
                    n956 = property on="表格" class="Tbl (严格)"() -> ("Selection Start"=w1205:T1)  [unwired: 2 in, 2 out]
                    n957 = Unbundle By Name(w1205) -> ("Row"=w1203:i32)
                    n958 = property on="表格" class="Tbl (严格)"() -> ("Value"=w1204:string[][])  [unwired: 2 in, 2 out]
                    n959 = Number To Decimal String(number=w1203) -> (decimal integer string=w1202:string)  [unwired: 1 in]
                    n960 = Index Array(array=w1204, index (row)=w1203, index (col)=0 ("禁用的索引 (列)")) -> (element=w1201:string)
                    n961 = String Subset(string=w1201, length (rest)=16 ("长度（剩余）")) -> (substring=w1200:string)  [unwired: 1 in]
                    n962 = property on="曲线42设置" class="Str"("Val(Sgnl)"=w1200) -> ()  [unwired: 2 in, 2 out]
                    n963 = invoke on="控件配置文件" class="Tbl (严格)" method="Set Cell Value"("X Index"=1 ("X索引"), "Y Index"=w1195, "Value"=w1202) -> ()  [unwired: 3 in, 6 out]
                    n964 = invoke on="控件配置文件" class="Tbl (严格)" method="Set Cell Value"("X Index"=0 ("X索引"), "Y Index"=w1195, "Value"=w1200) -> ()  [unwired: 3 in, 6 out]
                  }
                  frame "关联到曲线43" {
                    w1206 = T9 72 items=["刷新间隔", "波特率", "布尔1设置项", "布尔2设置项", "布尔3设置项", "布尔4设置项", "布尔5设置项", "布尔6设置项", "布尔7设置项", "布尔8设置项", "显控1设置", "显控2设置", "显控3设置", "显控4设置", "显控5设置", "显控6设置", "显控7设置", "显控8设置", "显控9设置", "显控10设置", "显控11设置", "显控12设置", "设控1设置", "设控2设置", "设控3设置", "设控4设置", "设控5设置", "设控6设置", "设控7设置", "设控8设置", "曲线1设置", "曲线2设置", "曲线3设置", "曲线4设置", "曲线5设置", "曲线6设置", "曲线7设置", "曲线8设置", "曲线9设置", "曲线10设置", "曲线11设置", "曲线12设置", "曲线13设置", "曲线14设置", "曲线15设置", "曲线16设置", "曲线17设置", "曲线18设置", "曲线19设置", "曲线20设置", "曲线21设置", "曲线22设置", "曲线23设置", "曲线24设置", "曲线25设置", "曲线26设置", "曲线27设置", "曲线28设置", "曲线29设置", "曲线30设置", "曲线31设置", "曲线32设置", "曲线33设置", "曲线34设置", "曲线35设置", "曲线36设置", "曲线37设置", "曲线38设置", "曲线39设置", "曲线40设置", "曲线41设置", "曲线42设置", "曲线43设置", "曲线44设置", "曲线45设置", "曲线46设置", "曲线47设置", "曲线48设置", "曲线49设置", "曲线50设置", "曲线51设置", "曲线52设置", "曲线53设置", "曲线54设置", "曲线55设置", "曲线56设置", "曲线57设置", "曲线58设置", "曲线59设置", "曲线60设置", "曲线61设置", "曲线62设置", "曲线63设置", "曲线64设置", "ID值", "数据模式"] ("DataInitDef")
                    n965 = property on="表格" class="Tbl (严格)"() -> ("Selection Start"=w1216:T1)  [unwired: 2 in, 2 out]
                    n966 = Unbundle By Name(w1216) -> ("Row"=w1214:i32)
                    n967 = property on="表格" class="Tbl (严格)"() -> ("Value"=w1215:string[][])  [unwired: 2 in, 2 out]
                    n968 = Number To Decimal String(number=w1214) -> (decimal integer string=w1213:string)  [unwired: 1 in]
                    n969 = Index Array(array=w1215, index (row)=w1214, index (col)=0 ("禁用的索引 (列)")) -> (element=w1212:string)
                    n970 = String Subset(string=w1212, length (rest)=16 ("长度（剩余）")) -> (substring=w1211:string)  [unwired: 1 in]
                    n971 = property on="曲线43设置" class="Str"("Val(Sgnl)"=w1211) -> ()  [unwired: 2 in, 2 out]
                    n972 = invoke on="控件配置文件" class="Tbl (严格)" method="Set Cell Value"("X Index"=1 ("X索引"), "Y Index"=w1206, "Value"=w1213) -> ()  [unwired: 3 in, 6 out]
                    n973 = invoke on="控件配置文件" class="Tbl (严格)" method="Set Cell Value"("X Index"=0 ("X索引"), "Y Index"=w1206, "Value"=w1211) -> ()  [unwired: 3 in, 6 out]
                  }
                  frame "关联到曲线44" {
                    w1217 = T9 73 items=["刷新间隔", "波特率", "布尔1设置项", "布尔2设置项", "布尔3设置项", "布尔4设置项", "布尔5设置项", "布尔6设置项", "布尔7设置项", "布尔8设置项", "显控1设置", "显控2设置", "显控3设置", "显控4设置", "显控5设置", "显控6设置", "显控7设置", "显控8设置", "显控9设置", "显控10设置", "显控11设置", "显控12设置", "设控1设置", "设控2设置", "设控3设置", "设控4设置", "设控5设置", "设控6设置", "设控7设置", "设控8设置", "曲线1设置", "曲线2设置", "曲线3设置", "曲线4设置", "曲线5设置", "曲线6设置", "曲线7设置", "曲线8设置", "曲线9设置", "曲线10设置", "曲线11设置", "曲线12设置", "曲线13设置", "曲线14设置", "曲线15设置", "曲线16设置", "曲线17设置", "曲线18设置", "曲线19设置", "曲线20设置", "曲线21设置", "曲线22设置", "曲线23设置", "曲线24设置", "曲线25设置", "曲线26设置", "曲线27设置", "曲线28设置", "曲线29设置", "曲线30设置", "曲线31设置", "曲线32设置", "曲线33设置", "曲线34设置", "曲线35设置", "曲线36设置", "曲线37设置", "曲线38设置", "曲线39设置", "曲线40设置", "曲线41设置", "曲线42设置", "曲线43设置", "曲线44设置", "曲线45设置", "曲线46设置", "曲线47设置", "曲线48设置", "曲线49设置", "曲线50设置", "曲线51设置", "曲线52设置", "曲线53设置", "曲线54设置", "曲线55设置", "曲线56设置", "曲线57设置", "曲线58设置", "曲线59设置", "曲线60设置", "曲线61设置", "曲线62设置", "曲线63设置", "曲线64设置", "ID值", "数据模式"] ("DataInitDef")
                    n974 = property on="表格" class="Tbl (严格)"() -> ("Selection Start"=w1227:T1)  [unwired: 2 in, 2 out]
                    n975 = Unbundle By Name(w1227) -> ("Row"=w1225:i32)
                    n976 = property on="表格" class="Tbl (严格)"() -> ("Value"=w1226:string[][])  [unwired: 2 in, 2 out]
                    n977 = Number To Decimal String(number=w1225) -> (decimal integer string=w1224:string)  [unwired: 1 in]
                    n978 = Index Array(array=w1226, index (row)=w1225, index (col)=0 ("禁用的索引 (列)")) -> (element=w1223:string)
                    n979 = String Subset(string=w1223, length (rest)=16 ("长度（剩余）")) -> (substring=w1222:string)  [unwired: 1 in]
                    n980 = property on="曲线44设置" class="Str"("Val(Sgnl)"=w1222) -> ()  [unwired: 2 in, 2 out]
                    n981 = invoke on="控件配置文件" class="Tbl (严格)" method="Set Cell Value"("X Index"=1 ("X索引"), "Y Index"=w1217, "Value"=w1224) -> ()  [unwired: 3 in, 6 out]
                    n982 = invoke on="控件配置文件" class="Tbl (严格)" method="Set Cell Value"("X Index"=0 ("X索引"), "Y Index"=w1217, "Value"=w1222) -> ()  [unwired: 3 in, 6 out]
                  }
                  frame "关联到曲线45" {
                    w1228 = T9 74 items=["刷新间隔", "波特率", "布尔1设置项", "布尔2设置项", "布尔3设置项", "布尔4设置项", "布尔5设置项", "布尔6设置项", "布尔7设置项", "布尔8设置项", "显控1设置", "显控2设置", "显控3设置", "显控4设置", "显控5设置", "显控6设置", "显控7设置", "显控8设置", "显控9设置", "显控10设置", "显控11设置", "显控12设置", "设控1设置", "设控2设置", "设控3设置", "设控4设置", "设控5设置", "设控6设置", "设控7设置", "设控8设置", "曲线1设置", "曲线2设置", "曲线3设置", "曲线4设置", "曲线5设置", "曲线6设置", "曲线7设置", "曲线8设置", "曲线9设置", "曲线10设置", "曲线11设置", "曲线12设置", "曲线13设置", "曲线14设置", "曲线15设置", "曲线16设置", "曲线17设置", "曲线18设置", "曲线19设置", "曲线20设置", "曲线21设置", "曲线22设置", "曲线23设置", "曲线24设置", "曲线25设置", "曲线26设置", "曲线27设置", "曲线28设置", "曲线29设置", "曲线30设置", "曲线31设置", "曲线32设置", "曲线33设置", "曲线34设置", "曲线35设置", "曲线36设置", "曲线37设置", "曲线38设置", "曲线39设置", "曲线40设置", "曲线41设置", "曲线42设置", "曲线43设置", "曲线44设置", "曲线45设置", "曲线46设置", "曲线47设置", "曲线48设置", "曲线49设置", "曲线50设置", "曲线51设置", "曲线52设置", "曲线53设置", "曲线54设置", "曲线55设置", "曲线56设置", "曲线57设置", "曲线58设置", "曲线59设置", "曲线60设置", "曲线61设置", "曲线62设置", "曲线63设置", "曲线64设置", "ID值", "数据模式"] ("DataInitDef")
                    n983 = property on="表格" class="Tbl (严格)"() -> ("Selection Start"=w1238:T1)  [unwired: 2 in, 2 out]
                    n984 = Unbundle By Name(w1238) -> ("Row"=w1236:i32)
                    n985 = property on="表格" class="Tbl (严格)"() -> ("Value"=w1237:string[][])  [unwired: 2 in, 2 out]
                    n986 = Number To Decimal String(number=w1236) -> (decimal integer string=w1235:string)  [unwired: 1 in]
                    n987 = Index Array(array=w1237, index (row)=w1236, index (col)=0 ("禁用的索引 (列)")) -> (element=w1234:string)
                    n988 = String Subset(string=w1234, length (rest)=16 ("长度（剩余）")) -> (substring=w1233:string)  [unwired: 1 in]
                    n989 = property on="曲线45设置" class="Str"("Val(Sgnl)"=w1233) -> ()  [unwired: 2 in, 2 out]
                    n990 = invoke on="控件配置文件" class="Tbl (严格)" method="Set Cell Value"("X Index"=1 ("X索引"), "Y Index"=w1228, "Value"=w1235) -> ()  [unwired: 3 in, 6 out]
                    n991 = invoke on="控件配置文件" class="Tbl (严格)" method="Set Cell Value"("X Index"=0 ("X索引"), "Y Index"=w1228, "Value"=w1233) -> ()  [unwired: 3 in, 6 out]
                  }
                  frame "关联到曲线46" {
                    w1239 = T9 75 items=["刷新间隔", "波特率", "布尔1设置项", "布尔2设置项", "布尔3设置项", "布尔4设置项", "布尔5设置项", "布尔6设置项", "布尔7设置项", "布尔8设置项", "显控1设置", "显控2设置", "显控3设置", "显控4设置", "显控5设置", "显控6设置", "显控7设置", "显控8设置", "显控9设置", "显控10设置", "显控11设置", "显控12设置", "设控1设置", "设控2设置", "设控3设置", "设控4设置", "设控5设置", "设控6设置", "设控7设置", "设控8设置", "曲线1设置", "曲线2设置", "曲线3设置", "曲线4设置", "曲线5设置", "曲线6设置", "曲线7设置", "曲线8设置", "曲线9设置", "曲线10设置", "曲线11设置", "曲线12设置", "曲线13设置", "曲线14设置", "曲线15设置", "曲线16设置", "曲线17设置", "曲线18设置", "曲线19设置", "曲线20设置", "曲线21设置", "曲线22设置", "曲线23设置", "曲线24设置", "曲线25设置", "曲线26设置", "曲线27设置", "曲线28设置", "曲线29设置", "曲线30设置", "曲线31设置", "曲线32设置", "曲线33设置", "曲线34设置", "曲线35设置", "曲线36设置", "曲线37设置", "曲线38设置", "曲线39设置", "曲线40设置", "曲线41设置", "曲线42设置", "曲线43设置", "曲线44设置", "曲线45设置", "曲线46设置", "曲线47设置", "曲线48设置", "曲线49设置", "曲线50设置", "曲线51设置", "曲线52设置", "曲线53设置", "曲线54设置", "曲线55设置", "曲线56设置", "曲线57设置", "曲线58设置", "曲线59设置", "曲线60设置", "曲线61设置", "曲线62设置", "曲线63设置", "曲线64设置", "ID值", "数据模式"] ("DataInitDef")
                    n992 = property on="表格" class="Tbl (严格)"() -> ("Selection Start"=w1249:T1)  [unwired: 2 in, 2 out]
                    n993 = Unbundle By Name(w1249) -> ("Row"=w1247:i32)
                    n994 = property on="表格" class="Tbl (严格)"() -> ("Value"=w1248:string[][])  [unwired: 2 in, 2 out]
                    n995 = Number To Decimal String(number=w1247) -> (decimal integer string=w1246:string)  [unwired: 1 in]
                    n996 = Index Array(array=w1248, index (row)=w1247, index (col)=0 ("禁用的索引 (列)")) -> (element=w1245:string)
                    n997 = String Subset(string=w1245, length (rest)=16 ("长度（剩余）")) -> (substring=w1244:string)  [unwired: 1 in]
                    n998 = property on="曲线46设置" class="Str"("Val(Sgnl)"=w1244) -> ()  [unwired: 2 in, 2 out]
                    n999 = invoke on="控件配置文件" class="Tbl (严格)" method="Set Cell Value"("X Index"=1 ("X索引"), "Y Index"=w1239, "Value"=w1246) -> ()  [unwired: 3 in, 6 out]
                    n1000 = invoke on="控件配置文件" class="Tbl (严格)" method="Set Cell Value"("X Index"=0 ("X索引"), "Y Index"=w1239, "Value"=w1244) -> ()  [unwired: 3 in, 6 out]
                  }
                  frame "关联到曲线47" {
                    w1250 = T9 76 items=["刷新间隔", "波特率", "布尔1设置项", "布尔2设置项", "布尔3设置项", "布尔4设置项", "布尔5设置项", "布尔6设置项", "布尔7设置项", "布尔8设置项", "显控1设置", "显控2设置", "显控3设置", "显控4设置", "显控5设置", "显控6设置", "显控7设置", "显控8设置", "显控9设置", "显控10设置", "显控11设置", "显控12设置", "设控1设置", "设控2设置", "设控3设置", "设控4设置", "设控5设置", "设控6设置", "设控7设置", "设控8设置", "曲线1设置", "曲线2设置", "曲线3设置", "曲线4设置", "曲线5设置", "曲线6设置", "曲线7设置", "曲线8设置", "曲线9设置", "曲线10设置", "曲线11设置", "曲线12设置", "曲线13设置", "曲线14设置", "曲线15设置", "曲线16设置", "曲线17设置", "曲线18设置", "曲线19设置", "曲线20设置", "曲线21设置", "曲线22设置", "曲线23设置", "曲线24设置", "曲线25设置", "曲线26设置", "曲线27设置", "曲线28设置", "曲线29设置", "曲线30设置", "曲线31设置", "曲线32设置", "曲线33设置", "曲线34设置", "曲线35设置", "曲线36设置", "曲线37设置", "曲线38设置", "曲线39设置", "曲线40设置", "曲线41设置", "曲线42设置", "曲线43设置", "曲线44设置", "曲线45设置", "曲线46设置", "曲线47设置", "曲线48设置", "曲线49设置", "曲线50设置", "曲线51设置", "曲线52设置", "曲线53设置", "曲线54设置", "曲线55设置", "曲线56设置", "曲线57设置", "曲线58设置", "曲线59设置", "曲线60设置", "曲线61设置", "曲线62设置", "曲线63设置", "曲线64设置", "ID值", "数据模式"] ("DataInitDef")
                    n1001 = property on="表格" class="Tbl (严格)"() -> ("Selection Start"=w1260:T1)  [unwired: 2 in, 2 out]
                    n1002 = Unbundle By Name(w1260) -> ("Row"=w1258:i32)
                    n1003 = property on="表格" class="Tbl (严格)"() -> ("Value"=w1259:string[][])  [unwired: 2 in, 2 out]
                    n1004 = Number To Decimal String(number=w1258) -> (decimal integer string=w1257:string)  [unwired: 1 in]
                    n1005 = Index Array(array=w1259, index (row)=w1258, index (col)=0 ("禁用的索引 (列)")) -> (element=w1256:string)
                    n1006 = String Subset(string=w1256, length (rest)=16 ("长度（剩余）")) -> (substring=w1255:string)  [unwired: 1 in]
                    n1007 = property on="曲线47设置" class="Str"("Val(Sgnl)"=w1255) -> ()  [unwired: 2 in, 2 out]
                    n1008 = invoke on="控件配置文件" class="Tbl (严格)" method="Set Cell Value"("X Index"=1 ("X索引"), "Y Index"=w1250, "Value"=w1257) -> ()  [unwired: 3 in, 6 out]
                    n1009 = invoke on="控件配置文件" class="Tbl (严格)" method="Set Cell Value"("X Index"=0 ("X索引"), "Y Index"=w1250, "Value"=w1255) -> ()  [unwired: 3 in, 6 out]
                  }
                  frame "关联到曲线48" {
                    w1261 = T9 77 items=["刷新间隔", "波特率", "布尔1设置项", "布尔2设置项", "布尔3设置项", "布尔4设置项", "布尔5设置项", "布尔6设置项", "布尔7设置项", "布尔8设置项", "显控1设置", "显控2设置", "显控3设置", "显控4设置", "显控5设置", "显控6设置", "显控7设置", "显控8设置", "显控9设置", "显控10设置", "显控11设置", "显控12设置", "设控1设置", "设控2设置", "设控3设置", "设控4设置", "设控5设置", "设控6设置", "设控7设置", "设控8设置", "曲线1设置", "曲线2设置", "曲线3设置", "曲线4设置", "曲线5设置", "曲线6设置", "曲线7设置", "曲线8设置", "曲线9设置", "曲线10设置", "曲线11设置", "曲线12设置", "曲线13设置", "曲线14设置", "曲线15设置", "曲线16设置", "曲线17设置", "曲线18设置", "曲线19设置", "曲线20设置", "曲线21设置", "曲线22设置", "曲线23设置", "曲线24设置", "曲线25设置", "曲线26设置", "曲线27设置", "曲线28设置", "曲线29设置", "曲线30设置", "曲线31设置", "曲线32设置", "曲线33设置", "曲线34设置", "曲线35设置", "曲线36设置", "曲线37设置", "曲线38设置", "曲线39设置", "曲线40设置", "曲线41设置", "曲线42设置", "曲线43设置", "曲线44设置", "曲线45设置", "曲线46设置", "曲线47设置", "曲线48设置", "曲线49设置", "曲线50设置", "曲线51设置", "曲线52设置", "曲线53设置", "曲线54设置", "曲线55设置", "曲线56设置", "曲线57设置", "曲线58设置", "曲线59设置", "曲线60设置", "曲线61设置", "曲线62设置", "曲线63设置", "曲线64设置", "ID值", "数据模式"] ("DataInitDef")
                    n1010 = property on="表格" class="Tbl (严格)"() -> ("Selection Start"=w1271:T1)  [unwired: 2 in, 2 out]
                    n1011 = Unbundle By Name(w1271) -> ("Row"=w1269:i32)
                    n1012 = property on="表格" class="Tbl (严格)"() -> ("Value"=w1270:string[][])  [unwired: 2 in, 2 out]
                    n1013 = Number To Decimal String(number=w1269) -> (decimal integer string=w1268:string)  [unwired: 1 in]
                    n1014 = Index Array(array=w1270, index (row)=w1269, index (col)=0 ("禁用的索引 (列)")) -> (element=w1267:string)
                    n1015 = String Subset(string=w1267, length (rest)=16 ("长度（剩余）")) -> (substring=w1266:string)  [unwired: 1 in]
                    n1016 = property on="曲线48设置" class="Str"("Val(Sgnl)"=w1266) -> ()  [unwired: 2 in, 2 out]
                    n1017 = invoke on="控件配置文件" class="Tbl (严格)" method="Set Cell Value"("X Index"=1 ("X索引"), "Y Index"=w1261, "Value"=w1268) -> ()  [unwired: 3 in, 6 out]
                    n1018 = invoke on="控件配置文件" class="Tbl (严格)" method="Set Cell Value"("X Index"=0 ("X索引"), "Y Index"=w1261, "Value"=w1266) -> ()  [unwired: 3 in, 6 out]
                  }
                  frame "关联到曲线49" {
                    w1272 = T9 78 items=["刷新间隔", "波特率", "布尔1设置项", "布尔2设置项", "布尔3设置项", "布尔4设置项", "布尔5设置项", "布尔6设置项", "布尔7设置项", "布尔8设置项", "显控1设置", "显控2设置", "显控3设置", "显控4设置", "显控5设置", "显控6设置", "显控7设置", "显控8设置", "显控9设置", "显控10设置", "显控11设置", "显控12设置", "设控1设置", "设控2设置", "设控3设置", "设控4设置", "设控5设置", "设控6设置", "设控7设置", "设控8设置", "曲线1设置", "曲线2设置", "曲线3设置", "曲线4设置", "曲线5设置", "曲线6设置", "曲线7设置", "曲线8设置", "曲线9设置", "曲线10设置", "曲线11设置", "曲线12设置", "曲线13设置", "曲线14设置", "曲线15设置", "曲线16设置", "曲线17设置", "曲线18设置", "曲线19设置", "曲线20设置", "曲线21设置", "曲线22设置", "曲线23设置", "曲线24设置", "曲线25设置", "曲线26设置", "曲线27设置", "曲线28设置", "曲线29设置", "曲线30设置", "曲线31设置", "曲线32设置", "曲线33设置", "曲线34设置", "曲线35设置", "曲线36设置", "曲线37设置", "曲线38设置", "曲线39设置", "曲线40设置", "曲线41设置", "曲线42设置", "曲线43设置", "曲线44设置", "曲线45设置", "曲线46设置", "曲线47设置", "曲线48设置", "曲线49设置", "曲线50设置", "曲线51设置", "曲线52设置", "曲线53设置", "曲线54设置", "曲线55设置", "曲线56设置", "曲线57设置", "曲线58设置", "曲线59设置", "曲线60设置", "曲线61设置", "曲线62设置", "曲线63设置", "曲线64设置", "ID值", "数据模式"] ("DataInitDef")
                    n1019 = property on="表格" class="Tbl (严格)"() -> ("Selection Start"=w1282:T1)  [unwired: 2 in, 2 out]
                    n1020 = Unbundle By Name(w1282) -> ("Row"=w1280:i32)
                    n1021 = property on="表格" class="Tbl (严格)"() -> ("Value"=w1281:string[][])  [unwired: 2 in, 2 out]
                    n1022 = Number To Decimal String(number=w1280) -> (decimal integer string=w1279:string)  [unwired: 1 in]
                    n1023 = Index Array(array=w1281, index (row)=w1280, index (col)=0 ("禁用的索引 (列)")) -> (element=w1278:string)
